vi "Read coatEnh.vi"(8 "error in":errorcluster, 11 "cPAS Data in":refnum<class "cPAS Data.lvclass">) -> (0 "error out":errorcluster, 2 "coatEnh":sgl, 3 "cPAS Data out":refnum<class "cPAS Data.lvclass">)   [LabVIEW 2015, in "cPAS Data.lvclass"]
uses:
  cPAS Data.lvclass
  cPAS Data.lvclass/cPAS Data.ctl
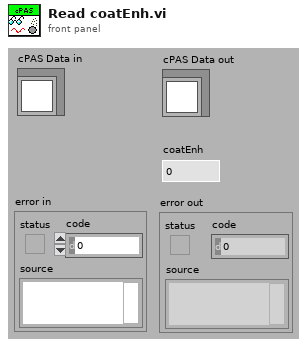
[diagram p1: front panel]
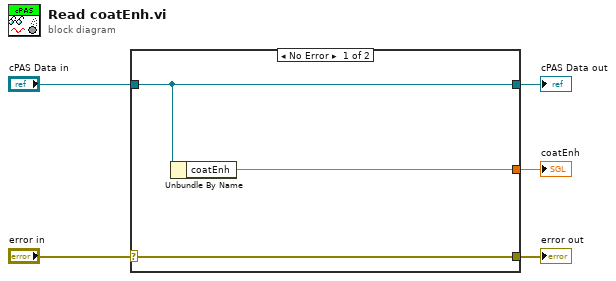
[diagram p0: block diagram]
diagram:
  n1 = case shown="No Error" "error in" {
    selector: "error in" -> [w8 w9]
    tunnel: [w8 w9] -> w4
    tunnel: [w7 w10] -> w2
    tunnel: "cPAS Data in" -> [w7 w10]
    tunnel: [w6 _] -> w1
    frame No Error {
      n2 = Unbundle By Name(w7) -> ("coatEnh"=w6:sgl)
    }
    frame Error {
    }
  }
  "error out" <- w4
  "cPAS Data out" <- w2
  "coatEnh" <- w1
